vi "Take Snapshot.vi"(8 "error in":errorcluster, 11 "Instruments in":refnum<class "Instruments.lvclass">) -> (0 "error out":errorcluster, 3 "Instruments out":refnum<class "Instruments.lvclass">)   [LabVIEW 2023, in "Instruments.lvlib" / "Instruments.lvclass"]
doc: "Use Snapshot Data to Generate a Group Separated Snapshot record. This eliminates nearly all the overhead in creating and removing a record group for snapshot data."
uses:
  Library/Instruments.lvclass
  C:/Users/Public/Documents/Development/builds/Engine/Engine.lvlibp/Project/Engine.lvclass
  C:/Users/Public/Documents/Development/builds/Engine/Actor Framework.lvlibp/1abvi3w/vi.lib/ActorFramework/Actor/Actor.lvclass
  Library/Instruments.lvclass/Instruments.ctl
  builds/Engine/Engine.lvlibp/Accessors/Read Report Queue.vi
  builds/Engine/Actor Framework.lvlibp/1abvi3w/vi.lib/ActorFramework/Actor/Read Actor Label.vi
  builds/Tools/QDMH.lvlibp/Private/Enqueue Bundled Element.vi
  builds/Tools/QDMH.lvlibp/QDMH.lvclass
  builds/Engine/Engine.lvlibp/Project/Engine.lvclass
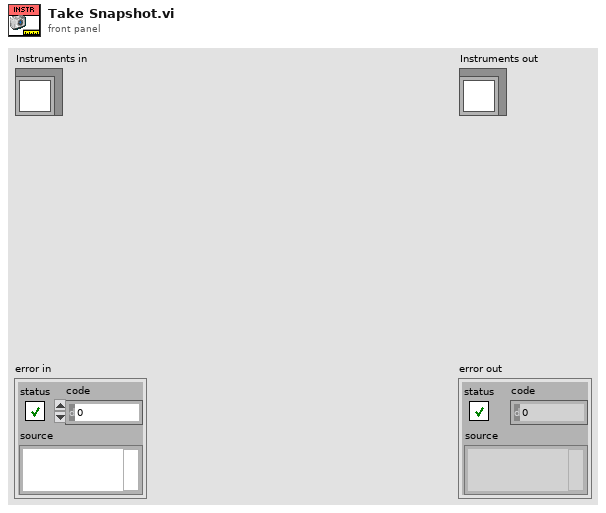
[diagram p1: front panel]
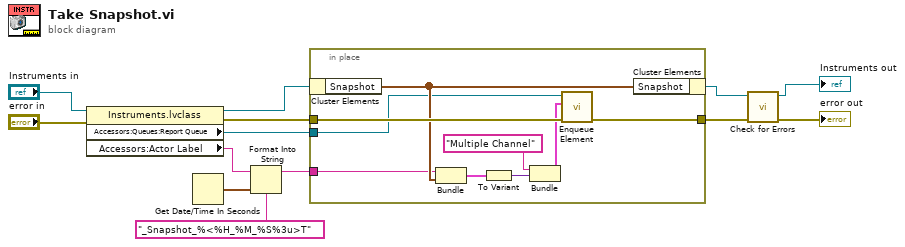
[diagram p0: block diagram]
diagram:
  n1 = property class="Instruments.lvclass"(reference="Instruments in", error in="error in") -> (reference out=w12:refnum<class "Instruments.lvclass">, error out=w11:errorcluster, "Accessors:Queues:Report Queue"=w13:refnum<class "QDMH.lvclass">, "Accessors:Actor Label"=w1:string)
  n2 = Get Date/Time In Seconds() -> (seconds since 1Jan1904=w4:timestamp)
  n3 = Format Into String(format string="_Snapshot_%<%H_%M_%S%3u>T", initial string=w1, w4) -> (resulting string=w3:string)  [unwired: 1 in, 1 out]
  n4 = in-place {
    in-place-border: w11 -> [w22]
    in-place-border: [w21] -> w10
    in-place-border: w13 -> [w15]
    in-place-border: w3 -> [w14]
    n5 = in-place-cluster #1(w12) -> ("Snapshot"=w16:waveform(dbl)[])
    n6 = Bundle(w14, "Snapshot"=w16) -> (w17:cluster{string, "Snapshot":waveform(dbl)[]})  [unwired: 1 in]
    n7 = To Variant(anything=w17) -> (Variant=w20:variant)
    n8 = Bundle("Multiple Channel", "Variant"=w20) -> (w19:cluster{string, "Variant":variant})  [unwired: 1 in]
    n9 = call-poly "Enqueue Element.vi"("error in"=w22, "element"=w19, "QDMH in"=w15) -> ("error out"=w21:errorcluster)  [unwired: 7 in, 1 out]
    n10 = in-place-cluster #1("Snapshot"=w16) -> (w9:refnum<class "Instruments.lvclass">)
  }
  n11 = call "Check for Errors.vi"("error in"=w10, "Engine in"=w9) -> ("error out"=→"error out":errorcluster, "Engine out"=→"Instruments out":refnum<class "Instruments.lvclass">)  [unwired: 8 in]
